vi "Query.vi"(0 "reference in":refnum<class "DatabaseInterface.lvclass">, 5 "Query":string, 7 "Timeout":i32=10000, 11 "error in (no error)":errorcluster) -> (4 "reference out":refnum<class "DatabaseInterface.lvclass">, 6 "Query Return":T1[](array[typedef]), 15 "error out":errorcluster)   [LabVIEW 2019, in "DatabaseInterface.lvclass"]
uses:
  DatabaseInterface.lvclass
  Database_Postgress_class/Query Return.ctl
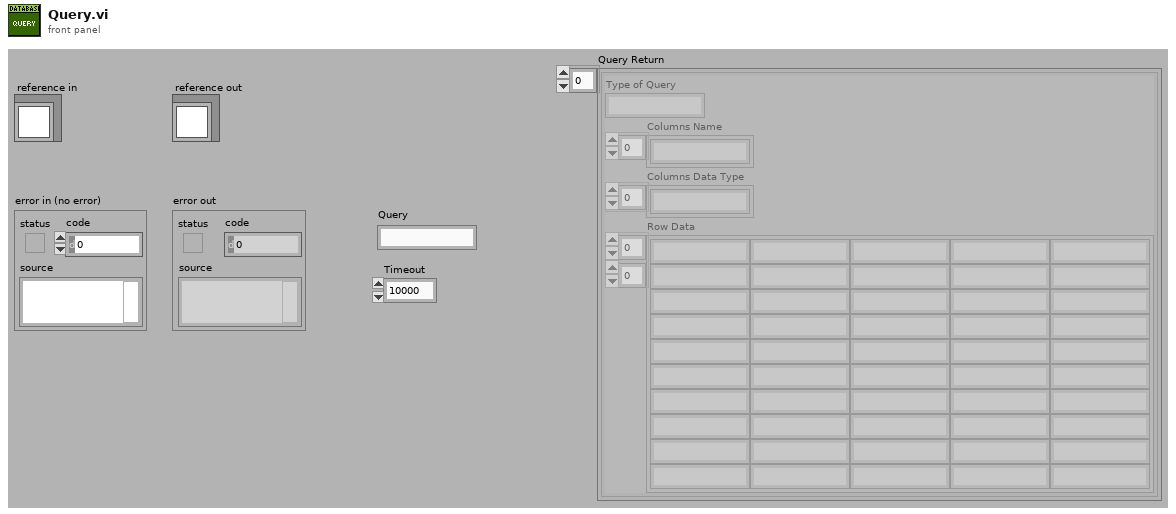
[diagram p1: front panel]
types:
  T1 = typedef "DatabaseInterface.lvclass/Query Return.ctl" = cluster{"Type of Query":string, "Columns Name":string[], "Columns Data Type":string[], "Row Data":string[][]}
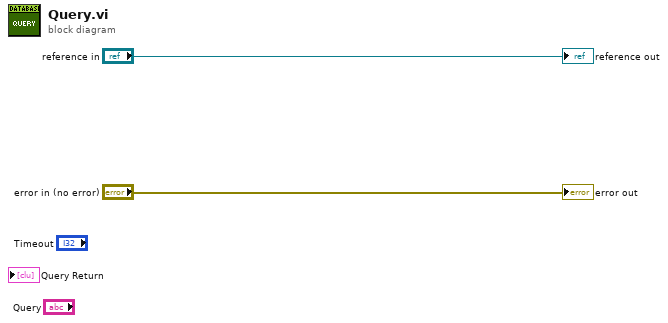
[diagram p0: block diagram]
diagram:
  "error out" <- "error in (no error)"
  "reference out" <- "reference in"
